vi "Init Default Views.vi"(6 "MainPane Actor":refnum<class "MainView.lvclass">, 8 "error in (no error)":errorcluster, 9 "CharmView Actor":refnum<class "CharmView.lvclass">, 10 "AppBarView Actor":refnum<class "AppBarView.lvclass">, 11 "DemoMain in":refnum<class "DemoMain.lvclass">) -> (0 "error out":errorcluster, 3 "DemoMain out":refnum<class "DemoMain.lvclass">)   [LabVIEW 2012, in "Win8uiDemo.lvlib" / "DemoMain.lvclass"]
doc: "Override this VI to provide default Actors for each SubView."
uses:
  DemoMain.lvclass
  Win8uiFramework/MainView.lvclass
  Win8uiFramework/CharmView.lvclass
  Win8uiFramework/AppBarView.lvclass
  SubPanel 3x3 View.lvclass
  DemoAppBar.lvclass
  Win8uiFramework/MainController.lvclass
  Win8uiFramework/MainController.lvclass/MainController.ctl
  DemoMain.lvclass/DemoMain.ctl
  <vilib>/ActorFramework/Message Enqueuer/Message Enqueuer.lvclass/Message Enqueuer.ctl
  Sensor Messages/Reschedule Acquire Msg/Reschedule Acquire Msg.lvclass/Reschedule Acquire Msg.ctl
  Win8uiFramework/Read MainPane Enqueuer.vi
  Read Sensor Enqueuers.vi
  Write GridView Enqueuer.vi
  Write GridView Capacity.vi
  <vilib>/ActorFramework/Message Enqueuer/Enqueue.vi
  <vilib>/ActorFramework/Message Priority Queue/Priority Enqueue.vi
  <vilib>/ActorFramework/Message Enqueuer/Message Enqueuer.lvclass
  Sensor Messages/Launch SmallView Msg/Launch SmallView Msg.lvclass
  Sensor Messages/Reschedule Acquire Msg/Reschedule Acquire Msg.lvclass
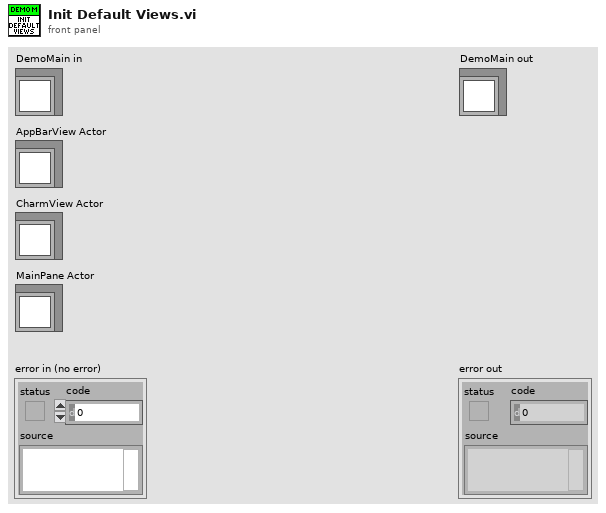
[diagram p1: front panel]
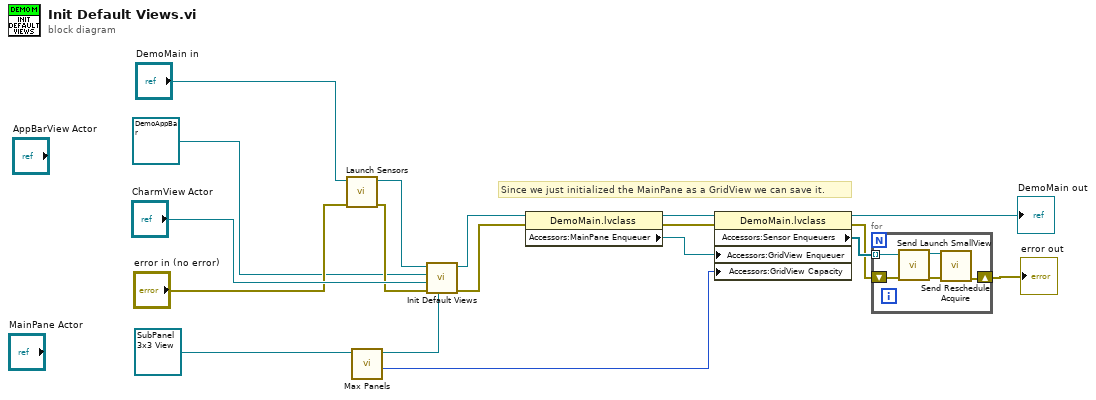
[diagram p0: block diagram]
diagram:
  # "Since we just initialized the MainPane as a GridView we can save it."
  n1 = call "Launch Sensors.vi"("error in (no error)"="error in (no error)", "DemoMain in"="DemoMain in") -> ("error out"=w14:errorcluster, "DemoMain out"=w16:refnum<class "DemoMain.lvclass">)  [unwired: 8 in]
  n2 = call-dynamic "Max Panels.vi"("SubPanel 3x3 View in"=refnum<class "SubPanel 3x3 View.lvclass"> refnum ("Win8uiDemo.lvlib:SubPanel 3x3 View.lvclass")) -> ("Max Panels"=w1:i32, "SubPanel 3x3 View out"=w2:refnum<class "SubPanel 3x3 View.lvclass">)  [unwired: 8 in, 1 out]
  n3 = call-parent "Init Default Views.vi"("MainPane Actor"=w2, "error in (no error)"=w14, "CharmView Actor"="CharmView Actor", "AppBarView Actor"=refnum<class "DemoAppBar.lvclass"> refnum ("Win8uiDemo.lvlib:DemoAppBar.lvclass"), "MainController in"=w16) -> ("error out"=w6:errorcluster, "MainController out"=w9:refnum<class "DemoMain.lvclass">)  [unwired: 5 in]
  n4 = property class="DemoMain.lvclass"(reference=w9, error in=w6) -> (reference out=w7:refnum<class "DemoMain.lvclass">, error out=w5:errorcluster, "Accessors:MainPane Enqueuer"=w4:refnum<class "Message Enqueuer.lvclass">)
  n5 = property class="DemoMain.lvclass"(reference=w7, error in=w5, "Accessors:GridView Enqueuer"=w4, "Accessors:GridView Capacity"=w1) -> (reference out=→"DemoMain out":refnum<class "DemoMain.lvclass">, error out=w12:errorcluster, "Accessors:Sensor Enqueuers"=w13:refnum<class "Message Enqueuer.lvclass">[])
  n6 = for {
    tunnel: w13 -> [w23] mode=indexing
    shift-right: [w19] -> w11
    shift-left: w12 -> [w22]
    n7 = call "Send Launch SmallView.vi"("error in (no error)"=w22, "Message Enqueuer"=w23) -> ("error out"=w21:errorcluster, "Message Enqueuer out"=w20:refnum<class "Message Enqueuer.lvclass">)  [unwired: 8 in]
    n8 = call "Send Reschedule Acquire.vi"("error in (no error)"=w21, "Message Enqueuer"=w20) -> ("error out"=w19:errorcluster)  [unwired: 8 in, 1 out]
  }
  "error out" <- w11
